vi "Power Down.vi"(8 "error in (no error)":errorcluster, 9 "Power Down Mode":T1, 10 "Channel Select":T2, 11 "DAC8552 in":refnum<class "LINX-DAC8552.lvclass">) -> (0 "error out":errorcluster, 3 "DAC8552 out":refnum<class "LINX-DAC8552.lvclass">)   [LabVIEW 2020, in "LINX-DAC8552.lvclass"]
doc: "Sends a power-down command to the specified channel(s). The channels can be configured to a specific resistance (1kOhm/100kOhm) or high-impedence."
uses:
  LINX-DAC8552.lvclass
  Channel Select.ctl
  Power Down Mode.ctl
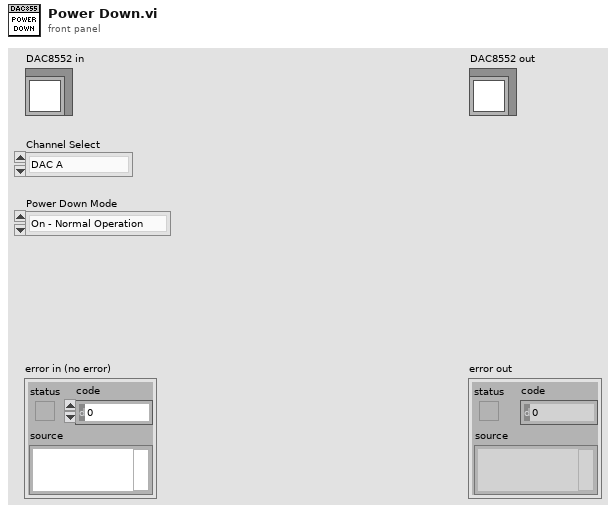
[diagram p1: front panel]
types:
  T1 = typedef "LINX-DAC8552.lvclass/Power Down Mode.ctl" = enum8{"On - Normal Operation", "Off - 1kOhm", "Off - 100kOhm", "Off - High Impedence"}
  T2 = typedef "LINX-DAC8552.lvclass/Channel Select.ctl" = enum8{"DAC A", "DAC B", "Both"}
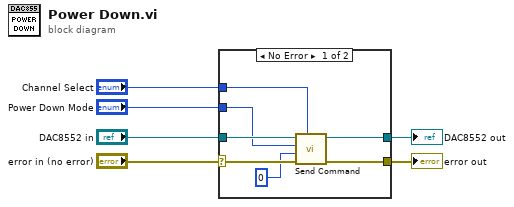
[diagram p0: block diagram]
diagram:
  n1 = case shown="No Error" "error in (no error)" {
    selector: "error in (no error)" -> [w11 w15]
    tunnel: [w10 w15] -> w5
    tunnel: [w12 w14] -> w3
    tunnel: "DAC8552 in" -> [w13 w14]
    tunnel: "Power Down Mode" -> [w9 _]
    tunnel: "Channel Select" -> [w8 _]
    frame No Error {
      n2 = call "Send Command.vi"("Channel Select"=w8, "error in (no error)"=w11, "Data"=u16 0, "Power Down Mode"=w9, "LINX-DAC8552 in"=w13) -> ("error out"=w10:errorcluster, "LINX-DAC8552 out"=w12:refnum<class "LINX-DAC8552.lvclass">)  [unwired: 5 in]
    }
    frame Error {
    }
  }
  "error out" <- w5
  "DAC8552 out" <- w3
